vi "Merge Wheel States.vi"(10 "wheel state with data":T1, 11 "wheel state with name":T1) -> (3 "merged wheel state":T1)   [LabVIEW 2017, in "NI_Robotics_Steering Frame.lvclass"]
doc: "Merges two wheel state clusters. The output contains the wheel name from the \"wheel state with name\" input and the numerical data from the \"wheel state with data\" input."
uses:
  <vilib>/robotics/Steering/Steering Frame/NI_Robotics_Steering Frame.lvclass
  <vilib>/robotics/Steering/Wheel/Wheel State.ctl
  <vilib>/robotics/Steering/Wheel/NI_Robotics_Wheel.lvclass
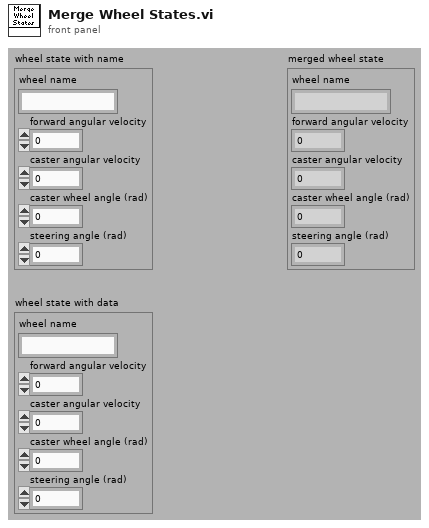
[diagram p1: front panel]
types:
  T1 = typedef "NI_Robotics_Wheel.lvclass/Wheel State.ctl" = cluster{"wheel name":string, "forward angular velocity":dbl, "caster angular velocity":dbl, "caster wheel angle (rad)":dbl, "steering angle (rad)":dbl}
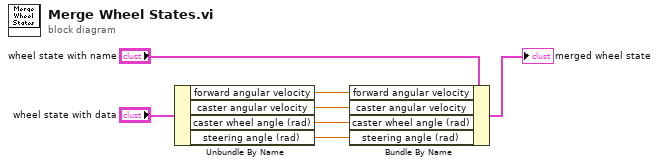
[diagram p0: block diagram]
diagram:
  n1 = Unbundle By Name("wheel state with data") -> ("forward angular velocity"=w4:dbl, "caster angular velocity"=w3:dbl, "caster wheel angle (rad)"=w2:dbl, "steering angle (rad)"=w1:dbl)
  n2 = Bundle By Name(cluster="wheel state with name", "forward angular velocity"=w4, "caster angular velocity"=w3, "caster wheel angle (rad)"=w2, "steering angle (rad)"=w1) -> (→"merged wheel state":T1)
